vi "Parallax PING Read Distance.vi"(8 "error in (no error)":errorcluster, 10 "Temperature (deg C)":dbl=25.0, 11 "myRIO DIO Channel":tag="C/DIO1") -> (0 "error out":errorcluster, 3 "Distance (m)":dbl)   [LabVIEW 2018]
doc: "Reads the distance in meters from the Parallax PING sensor located on the given pin.\n\nReturns -1 if the distance could not be read."
uses:
  <vilib>/myRIO/Instrument Drivers/Onboard IO/DIO/typedefs/DIO Reference.ctl
  <vilib>/myRIO/Common/Instrument Driver Framework/Utilities/typedefs/myRIO Generic Hardware Reference.ctl
  <vilib>/myRIO/Common/Instrument Driver Framework/Utilities/typedefs/Hardware Version Enum.ctl
  <vilib>/myRIO/Common/Instrument Driver Framework/Utilities/typedefs/myRIO v1.0 Reference.ctl
  <vilib>/myRIO/Common/Instrument Driver Framework/Utilities/typedefs/Generic FPGA Reference.ctl
  <vilib>/myRIO/Common/Instrument Driver Framework/myRIO v1.0/DIO/typedefs/DIO Channels List.ctl
  <vilib>/myRIO/Common/Instrument Driver Framework/myRIO v1.0/DIO/typedefs/DIO Channels Enum.ctl
  <vilib>/myRIO/Common/Instrument Driver Framework/myRIO v1.0/DIO/vis/myRIO v1.0 Close DIO.vi
  <vilib>/myRIO/Common/Instrument Driver Framework/myRIO v1.0/DIO/vis/myRIO v1.0 Unreserve DIO.vi
  <vilib>/myRIO/Common/Instrument Driver Framework/myRIO v1.0/DIO/vis/myRIO v1.0 Build MUX Configuration DIO.vi
  <vilib>/myRIO/Common/Instrument Driver Framework/myRIO v1.0/Resource Manager/vis/myRIO v1.0 Unreserve Channel List.vi
  <vilib>/myRIO/Common/Instrument Driver Framework/myRIO v1.0/Resource Manager/vis/myRIO v1.0 Create Configuration List.vi
  <vilib>/myRIO/Common/Instrument Driver Framework/myRIO v1.0/Resource Manager/vis/myRIO v1.0 Unreserve Channel.vi
  <vilib>/myRIO/Common/Instrument Driver Framework/myRIO v1.0/Resource Manager/vis/myRIO v1.0 Build Mutex Name.vi
  <vilib>/Utility/error.llb/Error Cluster From Error Code.vi
  <vilib>/myRIO/Common/Instrument Driver Framework/myRIO v1.0/DIO/vis/myRIO v1.0 Write DIO.vi
  <vilib>/myRIO/Common/Instrument Driver Framework/myRIO v1.0/DIO/vis/myRIO v1.0 Read DIO.vi
  <vilib>/myRIO/Common/Instrument Driver Framework/myRIO v1.0/DIO/vis/myRIO v1.0 Shutdown DIO.vi
  <vilib>/myRIO/Common/Instrument Driver Framework/myRIO v1.0/Resource Manager/vis/myRIO v1.0 Configure IO.vi
  <vilib>/myRIO/Common/Instrument Driver Framework/Utilities/vis/Configuration Manager.vi
  <vilib>/myRIO/Common/Instrument Driver Framework/Utilities/vis/IO Manager.vi
  <vilib>/myRIO/Common/Instrument Driver Framework/myRIO v1.0/myRIO v1.0 Close.vi
  <vilib>/myRIO/Instrument Drivers/Onboard IO/DIO/DIO.lvlib
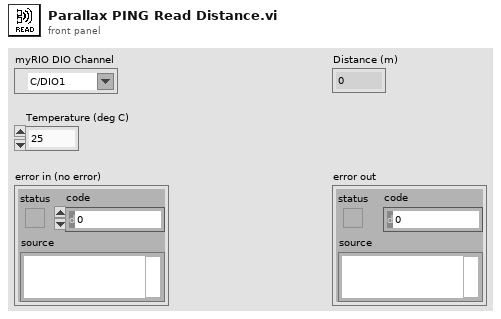
[diagram p1: front panel]
types:
  T1 = enum16{"Initialize", "Trigger pulse", "Wait for rising edge", "Wait for falling edge", "Calculate distance", "Stop"}
  T2 = typedef "DIO.lvlib/DIO Reference.ctl" = cluster{"myRIO Reference":T3, "DIO Channels List":T7}
  T3 = typedef "myRIO Generic Hardware Reference.ctl" = cluster{"myRIO Model":T4, "myRIO Hardware Reference":T5}
  T4 = typedef "Hardware Version Enum.ctl" = enum16{"Unknown", "myRIO-1900", "myRIO-1950", "roboRIO", "NI ELVIS RIO CM", "ELVIS III"}
  T5 = typedef "myRIO v1.0 Reference.ctl" = cluster{"Generic FPGA Reference":T6, "Allow multiple opens":bool}
  T6 = typedef "Generic FPGA Reference.ctl" = refnum<k20>
  T7 = typedef "DIO Channels List.ctl" = T8[]
  T8 = typedef "DIO Channels Enum.ctl" = enum16{"Not Connected", "C/DIO0", "C/DIO1", "C/DIO2", "C/DIO3", "C/DIO4", "C/DIO5", "C/DIO6", "C/DIO7", "A/DIO0", "A/DIO1", "A/DIO2", "A/DIO3", "A/DIO4", "A/DIO5", "A/DIO6", "A/DIO7", "A/DIO8", "A/DIO9", "A/DIO10", "A/DIO11", "A/DIO12", "A/DIO13", "A/DIO14", "A/DIO15", "A/DIO16", "A/DIO17", "A/DIO18", "A/DIO19", "B/DIO0", "B/DIO1", "B/DIO2", "B/DIO3", "B/DIO4", "B/DIO5", "B/DIO6", "B/DIO7", "B/DIO8", "B/DIO9", "B/DIO10", "B/DIO11", "B/DIO12", "B/DIO13", "B/DIO14", "B/DIO15", "B/DIO16", "B/DIO17", "B/DIO18", "B/DIO19", "LED0", "LED1", "LED2", "LED3", "Button0", "DIO/DIO0", "DIO/DIO1", "DIO/DIO2", "DIO/DIO3", "DIO/DIO4", "DIO/DIO5", "DIO/DIO6", "DIO/DIO7", "DIO/DIO8", "DIO/DIO9", "SPI/CS0", "SPI/CS1", "SPI/CS2", "SPI/CS3", "LED RADIO (Green)", "LED RADIO (Red)", "LED COMM (Green)", "LED COMM (Red)", "LED MODE (Green)", "LED MODE (Red)"}
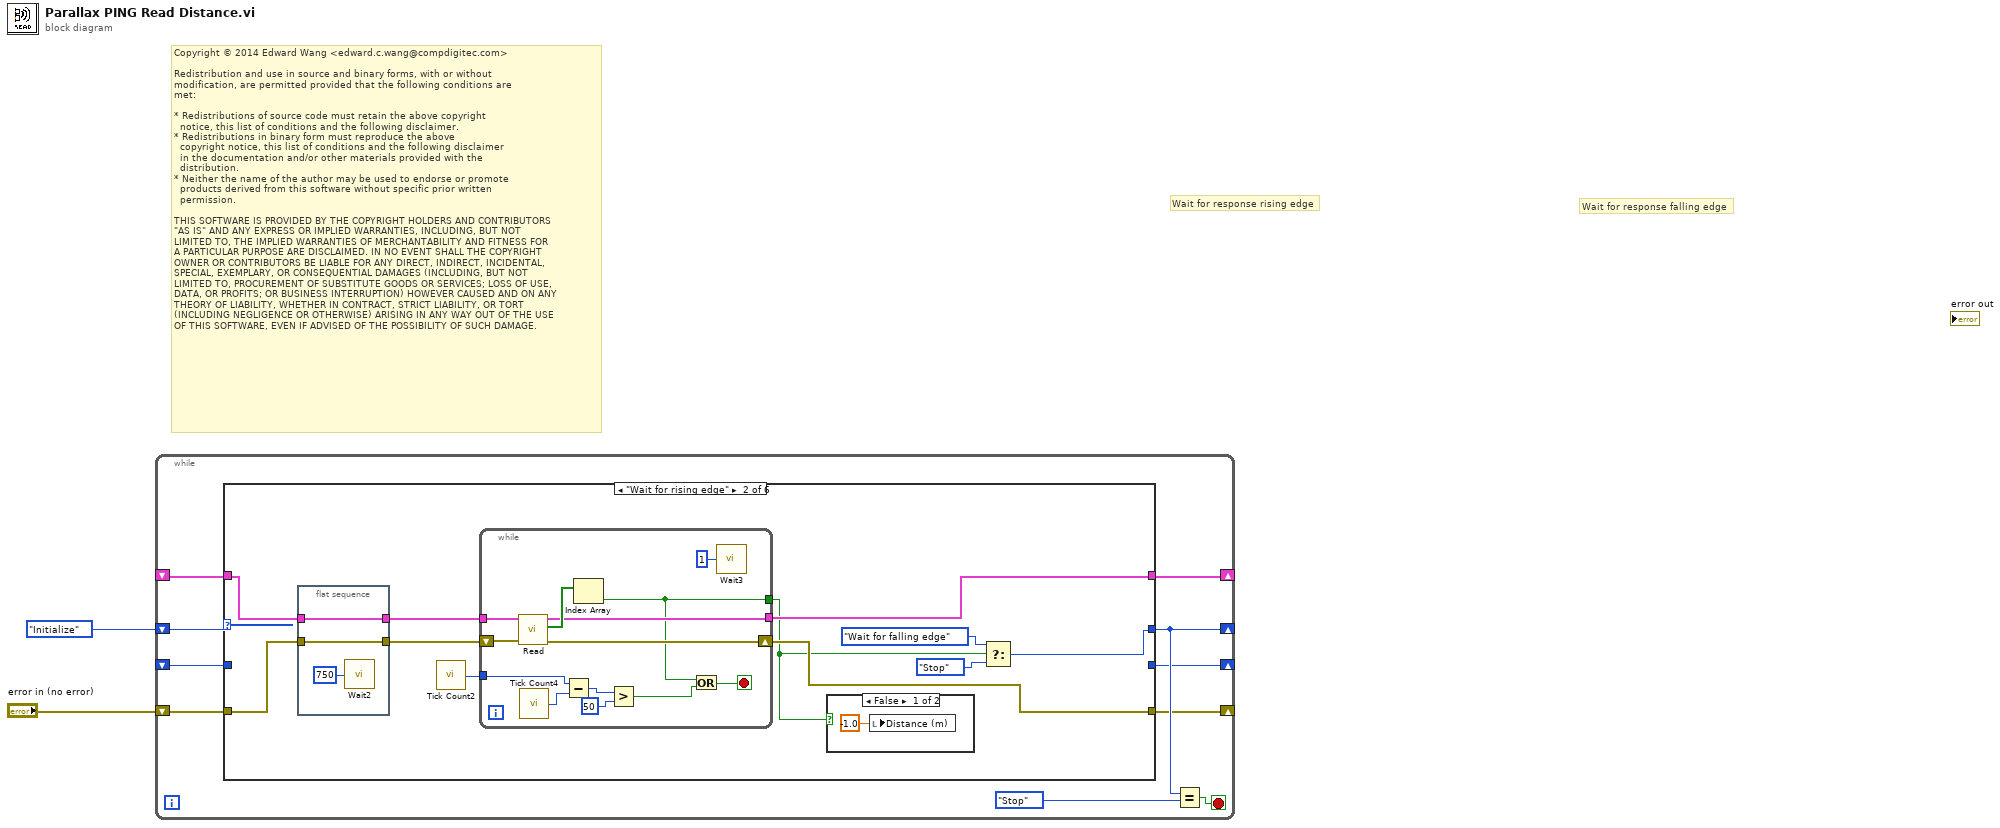
[diagram p0: block diagram]
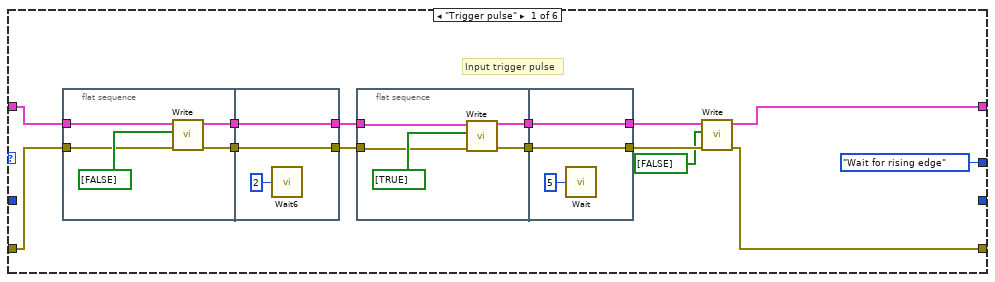
[diagram p2: hidden frame]
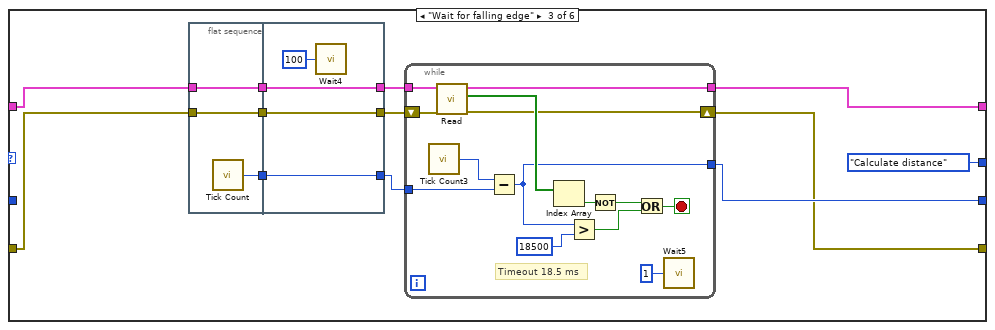
[diagram p4: hidden frame]
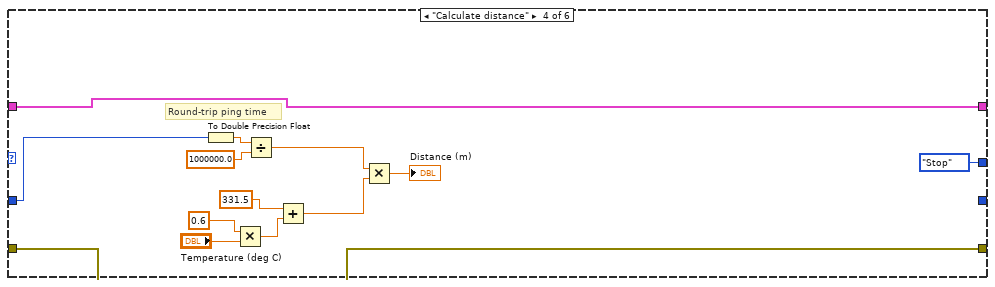
[diagram p5: hidden frame]
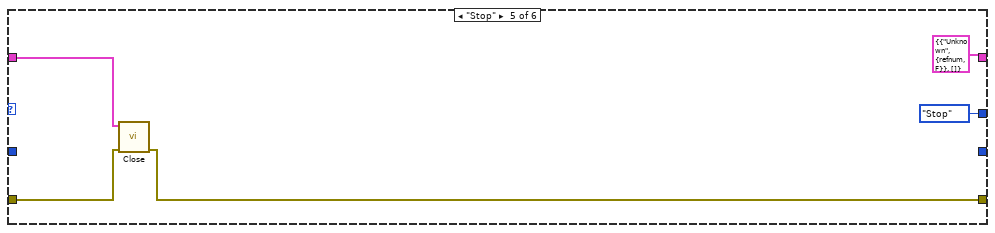
[diagram p6: hidden frame]
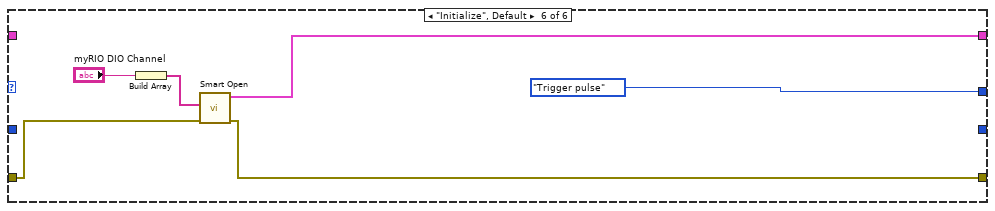
[diagram p7: hidden frame]
diagram:
  # "Copyright © 2014 Edward Wang <edward.c.wang@compdigitec.com>\n\nRedistribution and use in source and binary forms, with or without\nmodification, are permitted provided that the following conditions are\nmet:\n\n* Redistributions of source code must retain the above copyright\n  notice, this list of conditions and the following disclaimer.\n* Redistributions in binary form must reproduce the above\n  copyright notice, this list of conditions and the following disclaimer\n  in the documentation and/or other materials provided with the\n  distribution.\n* Neither the name of the author may be used to endorse or promote\n  products derived from this software without specific prior written\n  permission.\n\nTHIS SOFTWARE IS PROVIDED BY THE COPYRIGHT HOLDERS AND CONTRIBUTORS\n\"AS IS\" AND ANY EXPRESS OR IMPLIED WARRANTIES, INCLUDING, BUT NOT\nLIMITED TO, THE IMPLIED WARRANTIES OF MERCHANTABILITY AND FITNESS FOR\nA PARTICULAR PURPOSE ARE DISCLAIMED. IN NO EVENT SHALL THE COPYRIGHT\nOWNER OR CONTRIBUTORS BE LIABLE FOR ANY DIRECT, INDIRECT, INCIDENTAL,\nSPECIAL, EXEMPLARY, OR CONSEQUENTIAL DAMAGES (INCLUDING, BUT NOT\nLIMITED TO, PROCUREMENT OF SUBSTITUTE GOODS OR SERVICES; LOSS OF USE,\nDATA, OR PROFITS; OR BUSINESS INTERRUPTION) HOWEVER CAUSED AND ON ANY\nTHEORY OF LIABILITY, WHETHER IN CONTRACT, STRICT LIABILITY, OR TORT\n(INCLUDING NEGLIGENCE OR OTHERWISE) ARISING IN ANY WAY OUT OF THE USE\nOF THIS SOFTWARE, EVEN IF ADVISED OF THE POSSIBILITY OF SUCH DAMAGE."
  # "Wait for response falling edge"
  # "Wait for response rising edge"
  n1 = while {
    shift-right: [w11] -> _
    shift-left: T1."Initialize" -> [w10]
    shift-right: [w5] -> _
    shift-left: "error in (no error)" -> [w8]
    shift-right: [w7] -> _
    shift-left: _ -> [w6]
    shift-right: [w4] -> _
    shift-left: _ -> [w3]
    stop <- w12 stop-if-true
    n2 = case shown="\"Wait for rising edge\"" w10 {
      tunnel: [T1."Wait for rising edge" w47 T1."Calculate distance" ("y") T1."Stop" ("y") T1."Stop" ("y") T1."Trigger pulse"] -> w11
      tunnel: w8 -> [w17 w52 w75 w104 w120 w125]
      tunnel: [w15 w46 w74 w107 T2 {"myRIO Reference"={"myRIO Model"=enum."Unknown", "myRIO Hardware Reference"={"Generic FPGA Reference"=refnum, "Allow multiple opens"=FALSE}}, "DIO Channels List"=[]} ("DIO Ref Out") w124] -> w7
      tunnel: w6 -> [w16 w53 w76 w107 w119 _]
      tunnel: [w14 w45 w71 w104 w118 w123] -> w5
      tunnel: [_ _ w73 _ _ _] -> w4
      tunnel: w3 -> [_ _ _ w106 _ _]
      frame "Trigger pulse" {
        # "Input trigger pulse"
        n3 = flat-sequence {
          tunnel: [w30] -> w24
          tunnel: [w29] -> w23
          tunnel: w17 -> [w28]
          tunnel: w16 -> [w27]
          tunnel: [w33] -> w21
          tunnel: [w32] -> w22
          tunnel: w24 -> [w33]
          tunnel: w23 -> [w32]
          frame #0 {
            n4 = call <vilib>:"Write.vi"("error in (no error)"=w28, "Values"=bool[] [FALSE], "DIO Ref In"=w27) -> ("error out"=w29:errorcluster, "DIO Ref Out"=w30:T2)  [unwired: 6 in]
          }
          frame #1 {
            n5 = call "Wait6"("Count(uSec)"=u32 2) -> ()  [unwired: 1 out]
          }
        }
        n6 = flat-sequence {
          tunnel: [w38] -> w26
          tunnel: [w37] -> w25
          tunnel: w22 -> [w36]
          tunnel: w21 -> [w35]
          tunnel: [w41] -> w18
          tunnel: [w40] -> w20
          tunnel: w26 -> [w41]
          tunnel: w25 -> [w40]
          frame #0 {
            n7 = call <vilib>:"Write.vi"("error in (no error)"=w36, "Values"=bool[] [TRUE], "DIO Ref In"=w35) -> ("error out"=w37:errorcluster, "DIO Ref Out"=w38:T2)  [unwired: 6 in]
          }
          frame #1 {
            n8 = call "Wait"("Count(uSec)"=u32 5) -> ()  [unwired: 1 out]
          }
        }
        n9 = call <vilib>:"Write.vi"("error in (no error)"=w20, "Values"=bool[] [FALSE], "DIO Ref In"=w18) -> ("error out"=w14:errorcluster, "DIO Ref Out"=w15:T2)  [unwired: 6 in]
      }
      frame "Wait for rising edge" {
        n10 = flat-sequence {
          tunnel: w53 -> [w69]
          tunnel: w52 -> [w68]
          tunnel: [w69] -> w50
          tunnel: [w68] -> w51
          frame #0 {
            n11 = call "Wait2"("Count(uSec)"=u32 750) -> ()  [unwired: 1 out]
          }
        }
        n12 = call "Tick Count2"() -> ("Tick Count(uSec)"=w43:u32)
        n13 = while {
          tunnel: [w65] -> w46
          shift-right: [w63] -> w45
          shift-left: w51 -> [w64]
          tunnel: w43 -> [w60]
          tunnel: w50 -> [w62]
          tunnel: [w55] -> w44
          stop <- w57 stop-if-true
          n14 = call <vilib>:"Read.vi"("error in (no error)"=w64, "DIO Ref In"=w62) -> ("error out"=w63:errorcluster, "Values"=w66:bool[], "DIO Ref Out"=w65:T2)  [unwired: 7 in]
          n15 = call "Tick Count4"() -> ("Tick Count(uSec)"=w61:u32)
          n16 = Subtract(x=w60, y=w61) -> (x-y=w59:u32)
          n17 = Index Array(array=w66) -> (element=w55:bool)  [unwired: 1 in]
          n18 = Greater?(x=w59, y=u32 50) -> (0:w56:bool)
          n19 = Or(x=w55, y=w56) -> (x .or. y?=w57:bool)
          n20 = call "Wait3"("Count(uSec)"=u32 1) -> ()  [unwired: 1 out]
        }
        n21 = case shown="False" w44 {
          frame False {
            n22 = local write "Distance (m)"(-1.0 ("Distance (m)")) -> ()
          }
          frame True {
          }
        }
        n23 = Select(t=T1."Wait for falling edge", s=w44, f=T1."Stop" ("y")) -> (s? t:f=w47:T1)
      }
      frame "Wait for falling edge" {
        n24 = flat-sequence {
          tunnel: w76 -> [w99]
          tunnel: [w99] -> w82
          tunnel: [w98] -> w81
          tunnel: [w97] -> w80
          tunnel: w75 -> [w97]
          tunnel: [w102] -> w78
          tunnel: [w103] -> w79
          tunnel: w82 -> [w103]
          tunnel: w81 -> [w102]
          tunnel: w80 -> [w100]
          tunnel: [w100] -> w77
          frame #0 {
            n25 = call "Tick Count"() -> ("Tick Count(uSec)"=w98:u32)
          }
          frame #1 {
            n26 = call "Wait4"("Count(uSec)"=u32 100) -> ()  [unwired: 1 out]
          }
        }
        n27 = while {
          tunnel: w79 -> [w95]
          tunnel: w78 -> [w92]
          shift-right: [w86] -> w71
          shift-left: w77 -> [w87]
          tunnel: [w84] -> w74
          tunnel: [w83] -> w73
          stop <- w91 stop-if-true
          # "Timeout 18.5 ms"
          n28 = call "Tick Count3"() -> ("Tick Count(uSec)"=w85:u32)
          n29 = call <vilib>:"Read.vi"("error in (no error)"=w87, "DIO Ref In"=w95) -> ("error out"=w86:errorcluster, "Values"=w94:bool[], "DIO Ref Out"=w84:T2)  [unwired: 7 in]
          n30 = Subtract(x=w85, y=w92) -> (x-y=w83:u32)
          n31 = Index Array(array=w94) -> (element=w93:bool)  [unwired: 1 in]
          n32 = Greater?(x=w83, y=u32 18500) -> (0:w89:bool)
          n33 = Not(x=w93) -> (.not. x?=w90:bool)
          n34 = Or(x=w90, y=w89) -> (x .or. y?=w91:bool)
          n35 = call "Wait5"("Count(uSec)"=u32 1) -> ()  [unwired: 1 out]
        }
      }
      frame "Calculate distance" {
        # "Round-trip ping time"
        n36 = To Double Precision Float(number=w106) -> (double precision float=w112:dbl)
        n37 = Multiply(x=0.6, y="Temperature (deg C)") -> (x*y=w110:dbl)
        n38 = Divide(x=w112, y=1000000.0) -> (x/y=w114:dbl)
        n39 = Add(x=331.5, y=w110) -> (x+y=w115:dbl)
        n40 = Multiply(x=w114, y=w115) -> (x*y=→"Distance (m)":dbl)
      }
      frame "Stop" {
        n41 = call <vilib>:"Close.vi"("error in (no error)"=w120, "DIO Ref In"=w119) -> ("error out"=w118:errorcluster)  [unwired: 9 in]
      }
      frame "Initialize", Default {
        n42 = Build Array("myRIO DIO Channel") -> (w127:tag[])
        n43 = call <vilib>:"Smart Open.vi"("error in (no error)"=w125, "Channel Names"=w127) -> ("error out"=w123:errorcluster, "DIO Ref Out"=w124:T2)  [unwired: 8 in]
      }
    }
    n44 = Equal?(x=w11, y=T1."Stop") -> (x = y?=w12:bool)
  }
